vi "Ryans Script.vi"(6 "Variant in":variant, 7 "Shift Pressed?":bool, 8 "error in (no error)":errorcluster, 10 "QD Combo Box Ref":refnum<vi>, 11 "QD Launch VI Ref":refnum<vi>) -> (0 "error out":errorcluster, 4 "Variant out":variant)   [LabVIEW 2019]
doc: "Executes a series of plugin scripts using the Quick Drop Textbox to modify panel and diagram objects .\n\nGetting Started: 'Ctrl-Space' + type \"help\" + 'Ctrl-S'\n\nExample:\nChange a numeric control to U16, show radix in hex and hide the inc/dec buttons:\n1. On the front panel, select a numeric control\n2. 'Ctrl-Space' to open Quick Drop\n3. Type \"u16 rx hb\" in the Quick Drop Textbox\n4. 'Ctrl-S' to execute the script\n\nCreated by: Ryan Pacini\n\nDefault Shortcut - [S]"
uses:
  _Script/Script.lvlib
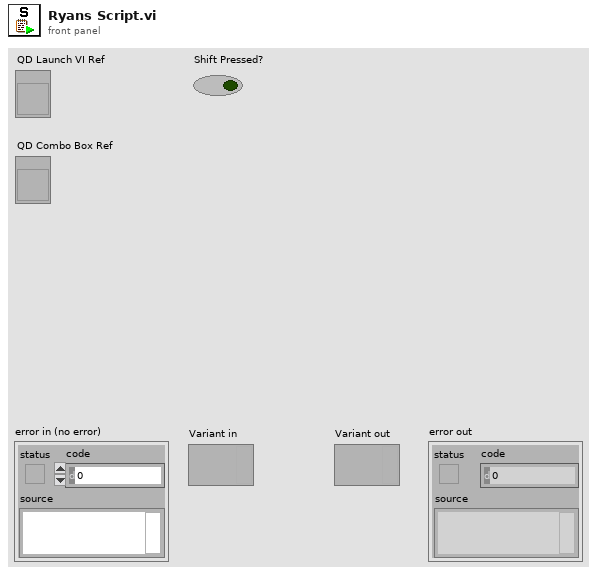
[diagram p1: front panel]
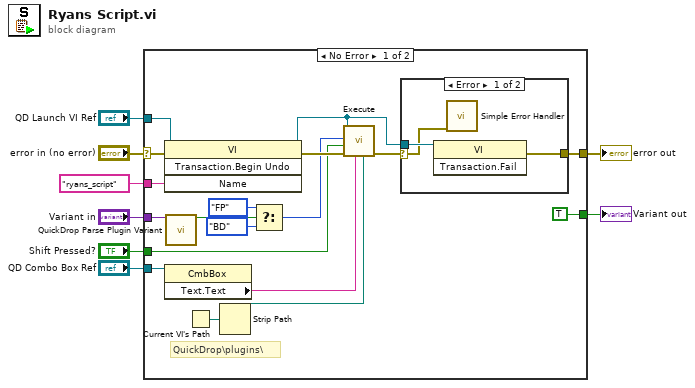
[diagram p0: block diagram]
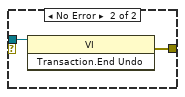
[diagram p2: hidden frame]
diagram:
  n1 = case shown="No Error" "error in (no error)" {
    selector: "error in (no error)" -> [w26 w32]
    tunnel: [w25 w32] -> w4
    tunnel: "QD Launch VI Ref" -> [w22 _]
    tunnel: "ryans_script" ("Undo Name") -> [w24 _]
    tunnel: [TRUE _] -> w5
    tunnel: "Variant in" -> [w21 _]
    tunnel: "QD Combo Box Ref" -> [w20 _]
    tunnel: "Shift Pressed?" -> [w13 _]
    frame No Error {
      # "QuickDrop\\plugins\\"
      n2 = invoke class="VI" method="Transaction.Begin Undo"(reference=w22, error in=w26, "Name"=w24) -> (reference out=w14:refnum<vi>, error out=w15:errorcluster)  [unwired: 1 in, 2 out]
      n3 = property class="CmbBox"(reference=w20) -> ("Text.Text"=w11:string)  [unwired: 1 in, 2 out]
      n4 = call <vilib>:"QuickDrop Parse Plugin Variant.vi"("QDKS Variant in"=w21) -> ("QD Launch VI Panel?"=w19:bool)  [unwired: 12 in, 2 out]
      n5 = Current VI's Path() -> (path=w10:path)
      n6 = Strip Path(path=w10) -> (stripped path=w9:path)  [unwired: 1 out]
      n7 = Select(t=enum8{"FP", "BD"}."FP" ("Panel"), s=w19, f=enum8{"FP", "BD"}."BD" ("Panel")) -> (s? t:f=w12:enum8{"FP", "BD"})
      n8 = call "Execute.vi"(4:w9, "QD Text"=w11, "error in (no error)"=w15, "Shift?"=w13, "Focus"=w12, "VI Refnum"=w14) -> ("error out"=w16:errorcluster)  [unwired: 5 in]
      n9 = case shown="Error" w16 {
        selector: w16 -> [w27 _]
        tunnel: w14 -> [w28 w30]
        tunnel: [w29 w31] -> w25
        frame Error {
          n10 = invoke class="VI" method="Transaction.Fail"(reference=w28) -> (error out=w29:errorcluster)  [unwired: 2 in, 2 out]
          n11 = call <vilib>:"Simple Error Handler.vi"("error in (no error)"=w27) -> ()  [unwired: 4 in, 5 out]
        }
        frame No Error {
          n12 = invoke class="VI" method="Transaction.End Undo"(reference=w30) -> (error out=w31:errorcluster)  [unwired: 2 in, 2 out]
        }
      }
    }
    frame Error {
    }
  }
  "error out" <- w4
  "Variant out" <- w5
